vi "Format LPC power string to mW.vi"(8 "error in (no error)":errorcluster, 10 "String":string) -> (0 "error out":errorcluster, 2 "power":dbl[unit])   [LabVIEW 2009, in "Laser Power Controller.lvclass"]
doc: "Takes an input string from the LPC (laser power controller) and returns a power reading in mW. If the string is formatted incorrectly or no power is found, it returns -1 as the power."
uses:
  Laser Power Controller.lvclass
  <vilib>/Utility/error.llb/DialogType.ctl
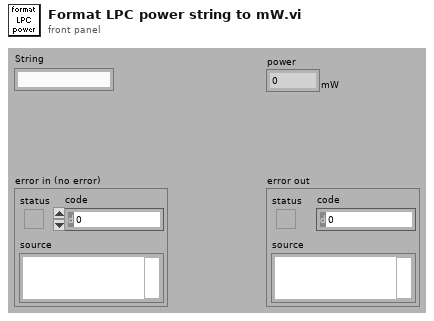
[diagram p1: front panel]
types:
  T1 = typedef "DialogType.ctl" = u16
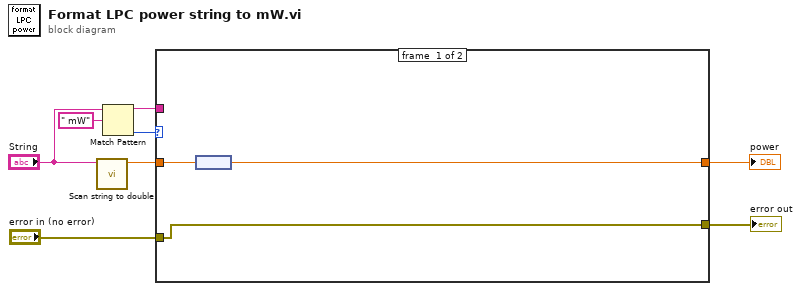
[diagram p0: block diagram]
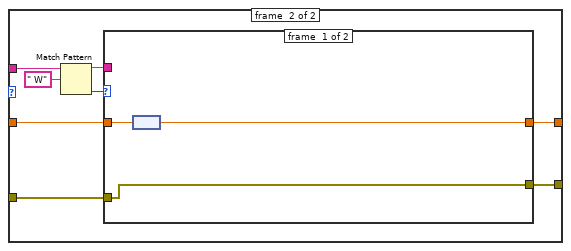
[diagram p2: hidden frame]
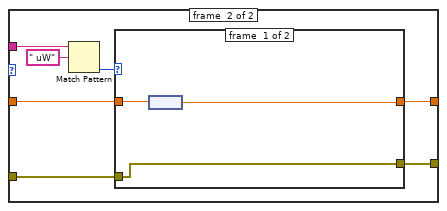
[diagram p3: hidden frame]
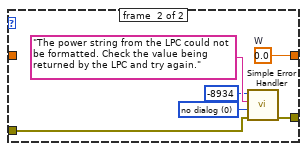
[diagram p4: hidden frame]
diagram:
  n1 = call "Scan string to double.vi"("String"="String") -> ("number"=w5:dbl)  [unwired: 1 in, 9 out]
  n2 = Match Pattern(string="String", regular expression=" mW") -> (before substring=w3:string, offset past match=w6:i32)  [unwired: 3 out]
  n3 = case shown="-1" w6 {
    tunnel: w5 -> [w11 w16]
    tunnel: [w10 w15] -> w4
    tunnel: w3 -> [_ w18]
    tunnel: "error in (no error)" -> [w9 w13]
    tunnel: [w9 w12] -> w1
    frame #0 {
      n4 = node(w11) -> (w10:dbl[unit])
    }
    frame #1 {
      n5 = Match Pattern(string=w18, regular expression=" W") -> (before substring=w14:string, offset past match=w17:i32)  [unwired: 3 out]
      n6 = case shown="-1" w17 {
        tunnel: w16 -> [w22 w26]
        tunnel: [w21 w25] -> w15
        tunnel: w14 -> [_ w28]
        tunnel: w13 -> [w20 w24]
        tunnel: [w20 w23] -> w12
        frame #0 {
          n7 = node(w22) -> (w21:dbl[unit])
        }
        frame #1 {
          n8 = Match Pattern(string=w28, regular expression=" uW") -> (offset past match=w27:i32)  [unwired: 4 out]
          n9 = case shown="-1" w27 {
            tunnel: w26 -> [w32 _]
            tunnel: [w31 w38] -> w25
            tunnel: w24 -> [w30 w34]
            tunnel: [w30 w33] -> w23
            frame #0 {
              n10 = node(w32) -> (w31:dbl[unit])
            }
            frame #1 {
              w37 = T1 0 items=["no dialog", "OK message", "continue or stop message", "OK message + warnings", "continue/stop + warnings"] ("type of dialog (OK msg:1)")
              w38 = dbl[unit] 0.0  # W
              n11 = call <vilib>:"Simple Error Handler.vi"("error code (no error:0)"=-8934, "error source (\" \")"="The power string from the LPC could not be formatted. Check the value being returned by the LPC and try again." ("error source (\" \")"), "type of dialog (OK msg:1)"=w37, "error in (no error)"=w34) -> ("error out"=w33:errorcluster)  [unwired: 5 out]
            }
          }
        }
      }
    }
  }
  "power" <- w4
  "error out" <- w1
